vi "WriteConfig.vi"(0 "reference in":refnum<class "NodeConfiguration.lvclass">, 2 "Config":T1, 5 "error in (no error)":errorcluster) -> (14 "reference out":refnum<class "NodeConfiguration.lvclass">, 19 "error out":errorcluster)   [LabVIEW 2014, in "NodeConfiguration.lvclass"]
uses:
  NodeConfiguration.lvclass
  Config.ctl
  <vilib>/Utility/config.llb/NI_LVConfig.lvlib
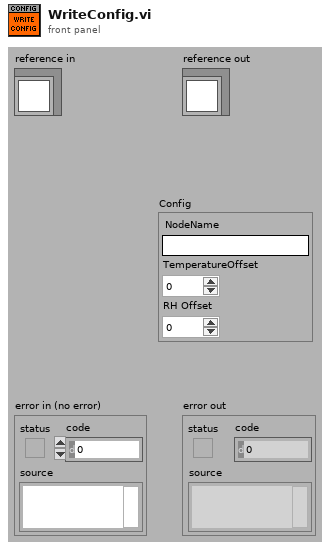
[diagram p1: front panel]
types:
  T1 = typedef "NodeConfiguration.lvclass/Config.ctl" = cluster{"NodeName":string, "TemperatureOffset":dbl, "RH Offset":dbl}
  T2 = typedef "NodeConfiguration.lvclass/ObjectAttributes.ctl" = cluster{"Config":T1, "ConfigFile":path}
  T3 = typedef "NI_LVConfig.lvlib/Config Data RefNum.ctl" = refnum<k1>
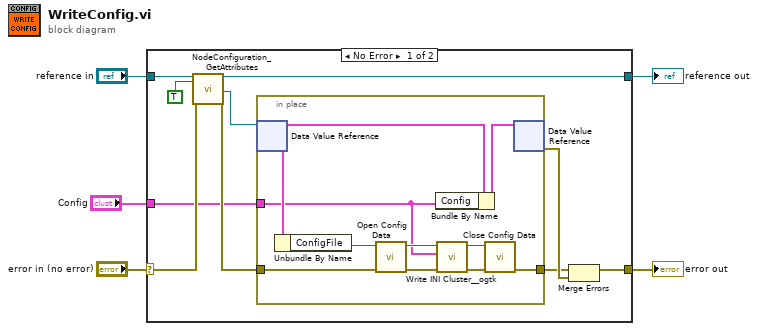
[diagram p0: block diagram]
diagram:
  n1 = case shown="No Error" "error in (no error)" {
    selector: "error in (no error)" -> [w12 w27]
    tunnel: [w14 w27] -> w4
    tunnel: [w10 w26] -> w2
    tunnel: "reference in" -> [w13 w26]
    tunnel: "Config" -> [w6 _]
    frame No Error {
      n2 = call "NodeConfiguration_GetAttributes.vi"("reference in"=w13, "OnlyGetDvrReference(False)"=TRUE, "error in (no error)"=w12) -> ("reference out"=w10:refnum<class "NodeConfiguration.lvclass">, "DataRef"=w11:refnum<data-value>, "error out"=w8:errorcluster)  [unwired: 13 in, 1 out]
      n3 = in-place {
        in-place-border: w8 -> [w23]
        in-place-border: [w21] -> w7
        in-place-border: w6 -> [w17]
        n4 = in-place-dvr #1(w11) -> (w24:T2)  [unwired: 1 out]
        n5 = Unbundle By Name(w24) -> ("ConfigFile"=w22:path)
        n6 = call <vilib>:"Open Config Data.vi"("error in (no error)"=w23, "configuration file path"=w22) -> ("error out"=w20:errorcluster, "refnum"=w19:T3)  [unwired: 7 in, 1 out]
        n7 = Bundle By Name(cluster=w24, "Config"=w17) -> (w25:T2)
        n8 = call <userlib>:"Write INI Cluster__ogtk.vi"("error in (no error)"=w20, "INI Fomatted Cluster"=w17, "refnum"=w19) -> ("error out"=w16:errorcluster, "dup refnum"=w18:T3)  [unwired: 7 in]
        n9 = call <vilib>:"Close Config Data.vi"("error in (no error)"=w16, "refnum"=w18) -> ("error out"=w21:errorcluster)  [unwired: 8 in, 1 out]
        n10 = in-place-dvr #1(w25) -> (w15:errorcluster)  [unwired: 1 out]
      }
      n11 = Merge Errors(w7, w15) -> (w14:errorcluster)
    }
    frame Error {
    }
  }
  "error out" <- w4
  "reference out" <- w2
